vi "Station Update.vi"(8 "error in (no error)":errorcluster, 9 "Instruments (none)":T1[](array[typedef]), 10 "Station Record (empty)":T2, 11 "Connection Refnum":T3) -> (0 "error out":errorcluster, 1 "Instruments on Station":T1[](array[typedef]), 2 "Station":T2, 3 "Connection Refnum":T3)   [LabVIEW 2011]
uses:
  Station Record.ctl
  Summitek EXT/ODBC/SQL Controls/Connection Refnum.ctl
  Instruments/Instrument Record.ctl
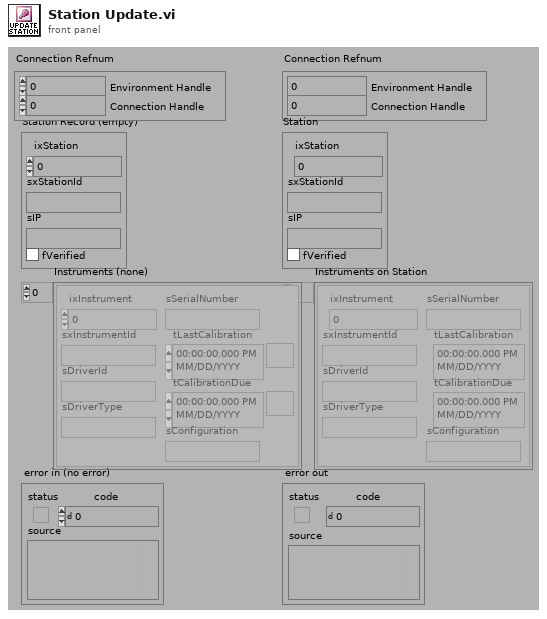
[diagram p1: front panel]
types:
  T1 = typedef "Instrument Record.ctl" = cluster{"ixInstrument":i32, "sxInstrumentId":string, "sDriverId":string, "sDriverType":string, "sSerialNumber":string, "tLastCalibration":timestamp, "tCalibrationDue":timestamp, "sConfiguration":string}
  T2 = typedef "Station Record.ctl" = cluster{"ixStation":i32, "sxStationId":string, "sIP":string, "fVerified":bool}
  T3 = typedef "Connection Refnum.ctl" = cluster{"Environment Handle":i32, "Connection Handle":i32}
  T4 = typedef "Statement Refnum.ctl" = cluster{"Statement Handle":i32, "Parameter Number":u16}
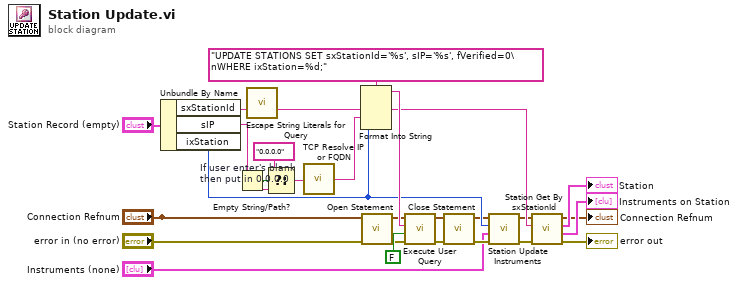
[diagram p0: block diagram]
diagram:
  w16 = "0.0.0.0"  # If user enter's blank then put in 0.0.0.0
  n1 = Unbundle By Name("Station Record (empty)") -> ("sxStationId"=w4:string, "sIP"=w13:string, "ixStation"=w10:i32)
  n2 = Empty String/Path?(string/path=w13) -> (empty?=w17:bool)
  n3 = call "Escape String Literals for Query.vi"("String"=w4) -> ("escaped String"=w3:string)  [unwired: 1 in, 13 out]
  n4 = Select(t=w16, s=w17, f=w13) -> (s? t:f=w8:string)
  n5 = call "TCP Resolve IP or FQDN.vi"("Machine (empty = this machine)"=w8) -> ("Resolved IP or FQDN"=w7:string)
  n6 = Format Into String(format string="UPDATE STATIONS SET sxStationId='%s', sIP='%s', fVerified=0\nWHERE ixStation=%d;" ("User Query"), w3, w7, w10) -> (resulting string=w20:string)  [unwired: 2 in, 1 out]
  n7 = call "Open Statement.vi"("error in (no error)"="error in (no error)", "Connection Refnum"="Connection Refnum") -> ("error out"=w19:errorcluster, "Statement Refnum"=w18:T4)  [unwired: 4 out]
  n8 = call "Execute User Query.vi"("error in (no error)"=w19, "Return Data? (f)"=FALSE, "User Query"=w20, "Statement Refnum"=w18) -> ("error out"=w23:errorcluster, "Statement Refnum"=w22:T4)  [unwired: 2 out]
  n9 = call "Close Statement.vi"("error in (no error)"=w23, "Statement Refnum"=w22) -> ("error out"=w12:errorcluster)  [unwired: 5 out]
  n10 = call "Station Update Instruments.vi"("error in (no error)"=w12, "Instruments on Station"="Instruments (none)", "Station KEY (0)"=w10, "Connection Refnum"="Connection Refnum") -> ("error out"=w11:errorcluster)  [unwired: 7 out]
  n11 = call "Station Get By sxStationId.vi"("error in (no error)"=w11, "sxStationId (\"\")"=w3, "Connection Refnum"="Connection Refnum") -> ("error out"=→"error out":errorcluster, "Instruments on Station"=→"Instruments on Station":T1[], "Station Record"=→"Station":T2, "Connection Refnum"=→"Connection Refnum":T3)  [unwired: 5 out]
